vi "Read Frequency and Amplitude.vi"(0 "Microwave.lvclass in":refnum<class "Microwave.lvclass">, 11 "error in (no error)":errorcluster) -> (4 "Microwave.lvclass out":refnum<class "Microwave.lvclass">, 6 "Frequency":dbl[unit], 8 "Amplitude (dBm)":dbl, 10 "rf on?":bool, 15 "error out":errorcluster)   [LabVIEW 2009, in "Microwave.lvclass"]
uses:
  Microwave.lvclass
  Microwave.lvclass/Microwave.ctl
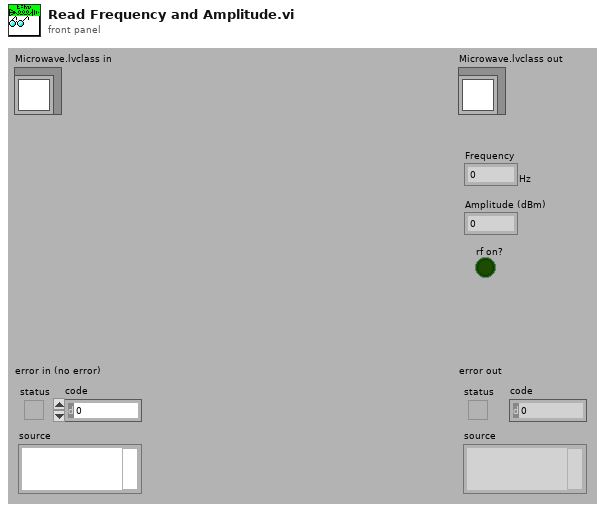
[diagram p1: front panel]
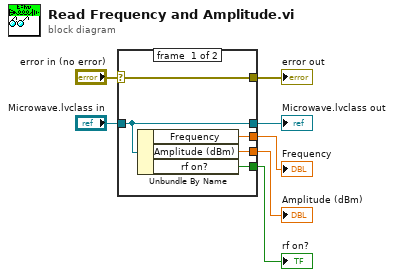
[diagram p0: block diagram]
diagram:
  n1 = case shown="No Error" "error in (no error)" {
    selector: "error in (no error)" -> [w12 w13]
    tunnel: [w12 w13] -> w6
    tunnel: [w11 w14] -> w4
    tunnel: "Microwave.lvclass in" -> [w11 w14]
    tunnel: [w10 _] -> w3
    tunnel: [w9 _] -> w2
    tunnel: [w8 _] -> w1
    frame #0 {
      n2 = Unbundle By Name(w11) -> ("Frequency"=w9:dbl[unit], "Amplitude (dBm)"=w10:dbl, "rf on?"=w8:bool)
    }
    frame #1 {
    }
  }
  "error out" <- w6
  "Microwave.lvclass out" <- w4
  "Amplitude (dBm)" <- w3
  "Frequency" <- w2
  "rf on?" <- w1
